vi "SetupProcess.vi"(8 "error in (no error)":errorcluster, 10 "SetupData":string, 11 "ScopeAA in":refnum<class "ScopeAA.lvclass">) -> (0 "error out":errorcluster, 2 "Type":string, 3 "ScopeAA out":refnum<class "ScopeAA.lvclass">)   [LabVIEW 2025, in "ScopeAA.lvclass"]
uses:
  ScopeAA.lvclass
  ScopeAA.lvclass/ScopeAA.ctl
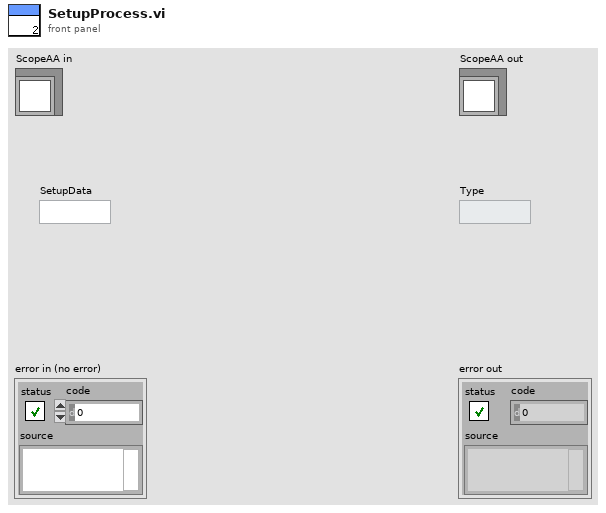
[diagram p1: front panel]
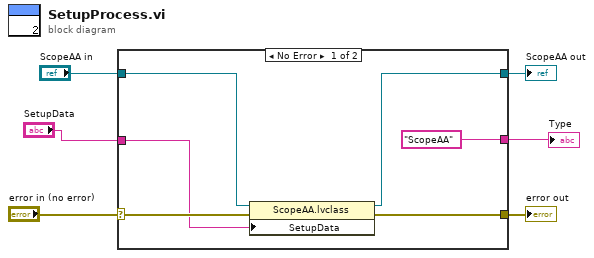
[diagram p0: block diagram]
diagram:
  n1 = case shown="No Error" "error in (no error)" {
    selector: "error in (no error)" -> [w12 w14]
    tunnel: [w11 w14] -> w6
    tunnel: [w9 w13] -> w5
    tunnel: "ScopeAA in" -> [w10 w13]
    tunnel: "SetupData" -> [w8 _]
    tunnel: ["ScopeAA" _] -> w1
    frame No Error {
      n2 = property class="ScopeAA.lvclass"(reference=w10, error in=w12, "SetupData"=w8) -> (reference out=w9:refnum<class "ScopeAA.lvclass">, error out=w11:errorcluster)
    }
    frame Error {
    }
  }
  "error out" <- w6
  "ScopeAA out" <- w5
  "Type" <- w1
